vi "UHR-Fleezers Control (host) - Lorentz v2.vi"() -> ()   [LabVIEW 2014] (continued)
        n3462 = call-poly <vilib>:"Mean.vi"("X"=w5310) -> ("mean"=w5257:dbl)  [unwired: 1 out]
        n3463 = call-poly <vilib>:"Mean.vi"("X"=w5266) -> ("mean"=w5250:dbl)  [unwired: 1 out]
        n3464 = call-poly <vilib>:"Mean.vi"("X"=w5268) -> ("mean"=w5255:dbl)  [unwired: 1 out]
        n3465 = call-poly <vilib>:"Mean.vi"("X"=w5267) -> ("mean"=w5253:dbl)  [unwired: 1 out]
        n3466 = Initialize Array(1.0 ("element"), w5238) -> (w5234:dbl[])
        n3467 = Initialize Array(1.0 ("element"), w5219) -> (w5215:dbl[])
        n3468 = Initialize Array(1.0 ("element"), w5260) -> (w5251:dbl[])
        n3469 = Multiply(x=w5234, y=w5235) -> (x*y=w5236:dbl[])
        n3470 = Multiply(x=w5215, y=w5216) -> (x*y=w5217:dbl[])
        n3471 = Multiply(x=w5251, y=w5257) -> (x*y=w5258:dbl[])
        n3472 = Multiply(x=w5251, y=w5253) -> (x*y=w5254:dbl[])
        n3473 = Multiply(x=w5251, y=w5255) -> (x*y=w5256:dbl[])
        n3474 = Multiply(x=w5251, y=w5250) -> (x*y=w5252:dbl[])
        n3475 = Build Array (concatenate)(w5244, w5236) -> (w5246:dbl[])
        n3476 = Build Array (concatenate)(w5225, w5217) -> (w5227:dbl[])
        n3477 = Build Array (concatenate)(w5310, w5258) -> (w5319:dbl[])
        n3478 = Build Array (concatenate)(w5266, w5252) -> (w5314:dbl[])
        n3479 = Build Array (concatenate)(w5268, w5256) -> (w5318:dbl[])
        n3480 = Build Array (concatenate)(w5267, w5254) -> (w5317:dbl[])
        n3481 = Reshape Array(w5246, w5200, w5201) -> (w5242:dbl[][])
        n3482 = Reshape Array(w5227, w5200, w5201) -> (w5223:dbl[][])
        n3483 = Reshape Array(w5319, w5200, w5201) -> (w5297:dbl[][])
        n3484 = Reshape Array(w5314, w5200, w5201) -> (w5280:dbl[][])
        n3485 = Reshape Array(w5318, w5200, w5201) -> (w5272:dbl[][])
        n3486 = Reshape Array(w5317, w5200, w5201) -> (w5287:dbl[][])
        n3487 = Array Subset(array=w5242, index (col)=0 ("index"), length (col)=w5199) -> (w5241:dbl[][])  [unwired: 2 in]
        n3488 = Array Subset(array=w5242, index (col)=w5199) -> (w5239:dbl[][])  [unwired: 3 in]
        n3489 = Array Subset(array=w5223, index (col)=0 ("index"), length (col)=w5199) -> (w5222:dbl[][])  [unwired: 2 in]
        n3490 = Array Subset(array=w5223, index (col)=w5199) -> (w5220:dbl[][])  [unwired: 3 in]
        n3491 = Array Subset(array=w5287, index (col)=0 ("index"), length (col)=w5199) -> (w5292:dbl[][])  [unwired: 2 in]
        n3492 = Array Subset(array=w5287, index (col)=w5199) -> (w5290:dbl[][])  [unwired: 3 in]
        n3493 = Array Subset(array=w5297, index (col)=0 ("index"), length (col)=w5199) -> (w5296:dbl[][])  [unwired: 2 in]
        n3494 = Array Subset(array=w5297, index (col)=w5199) -> (w5294:dbl[][])  [unwired: 3 in]
        n3495 = Array Subset(array=w5272, index (col)=0 ("index"), length (col)=w5199) -> (w5278:dbl[][])  [unwired: 2 in]
        n3496 = Array Subset(array=w5272, index (col)=w5199) -> (w5276:dbl[][])  [unwired: 3 in]
        n3497 = Array Subset(array=w5280, index (col)=0 ("index"), length (col)=w5199) -> (w5285:dbl[][])  [unwired: 2 in]
        n3498 = Array Subset(array=w5280, index (col)=w5199) -> (w5283:dbl[][])  [unwired: 3 in]
        n3499 = for {
          tunnel: w5241 -> [w5328] mode=indexing
          tunnel: [w5327] -> w5240 mode=indexing
          workers-P: _ -> [_]
          n3500 = Reverse 1D Array(array=w5328) -> (reversed array=w5327:dbl[])
        }
        n3501 = for {
          tunnel: w5222 -> [w5326] mode=indexing
          tunnel: [w5325] -> w5221 mode=indexing
          workers-P: _ -> [_]
          n3502 = Reverse 1D Array(array=w5326) -> (reversed array=w5325:dbl[])
        }
        n3503 = for {
          tunnel: w5292 -> [w5334] mode=indexing
          tunnel: [w5333] -> w5291 mode=indexing
          workers-P: _ -> [_]
          n3504 = Reverse 1D Array(array=w5334) -> (reversed array=w5333:dbl[])
        }
        n3505 = for {
          tunnel: w5296 -> [w5336] mode=indexing
          tunnel: [w5335] -> w5295 mode=indexing
          workers-P: _ -> [_]
          n3506 = Reverse 1D Array(array=w5336) -> (reversed array=w5335:dbl[])
        }
        n3507 = for {
          tunnel: w5278 -> [w5330] mode=indexing
          tunnel: [w5329] -> w5277 mode=indexing
          workers-P: _ -> [_]
          n3508 = Reverse 1D Array(array=w5330) -> (reversed array=w5329:dbl[])
        }
        n3509 = for {
          tunnel: w5285 -> [w5332] mode=indexing
          tunnel: [w5331] -> w5284 mode=indexing
          workers-P: _ -> [_]
          n3510 = Reverse 1D Array(array=w5332) -> (reversed array=w5331:dbl[])
        }
        n3511 = Index Array(array=w5297, index (row)=0) -> (element=→"Waveform Graph":dbl[])  [unwired: 1 in]
        n3512 = Add(x=w5240, y=w5239) -> (x+y=w5232:dbl[][])
        n3513 = Add(x=w5221, y=w5220) -> (x+y=w5213:dbl[][])
        n3514 = Add(x=w5291, y=w5290) -> (x+y=w5289:dbl[][])
        n3515 = Add(x=w5295, y=w5294) -> (x+y=w5271:dbl[][])
        n3516 = Add(x=w5277, y=w5276) -> (x+y=w5275:dbl[][])
        n3517 = Add(x=w5284, y=w5283) -> (x+y=w5282:dbl[][])
        n3518 = Divide(x=w5275, y=2) -> (x/y=w5273:dbl[][])
        n3519 = Divide(x=w5289, y=2) -> (x/y=w5179:dbl[][])
        n3520 = To Single Precision Float(number=w5271) -> (single precision float=w5192:sgl[][])
        n3521 = To Single Precision Float(number=w5232) -> (single precision float=w5175:sgl[][])
        n3522 = To Single Precision Float(number=w5213) -> (single precision float=w5168:sgl[][])
        n3523 = Divide(x=w5282, y=2) -> (x/y=w5181:dbl[][])
        n3524 = Transpose 2D Array(2D array=w5273) -> (transposed array=→"Data map":dbl[][])
        n3525 = To Single Precision Float(number=w5179) -> (single precision float=w5185:sgl[][])
        n3526 = To Single Precision Float(number=w5181) -> (single precision float=w5182:sgl[][])
        n3527 = call "IMAQ ArrayToImage"("Image Pixels (Float)"=w5192, "Image"=w5230) -> ("Image Out"=w5194:T2)  [unwired: 8 in, 1 out]
        n3528 = call "IMAQ ArrayToImage"("Image Pixels (Float)"=w5175, "Image"=w5229) -> ("Image Out"=w5177:T2)  [unwired: 8 in, 1 out]
        n3529 = call "IMAQ ArrayToImage"("Image Pixels (Float)"=w5168, "Image"=w5210) -> ("Image Out"=w5170:T2)  [unwired: 8 in, 1 out]
        n3530 = call "IMAQ ArrayToImage"("Image Pixels (Float)"=w5185, "Image"=w5211) -> ("Image Out"=w5187:T2)  [unwired: 8 in, 1 out]
        n3531 = call "IMAQ Symmetry"("Type of Symmetry"=w5193, "Image Src"=w5194) -> ("Image Dst Out"=w5190:T2)  [unwired: 3 in, 1 out]
        n3532 = call "IMAQ ArrayToImage"("Image Pixels (Float)"=w5182, "Image"=w5212) -> ("Image Out"=w5184:T2)  [unwired: 8 in, 1 out]
        n3533 = call "IMAQ Symmetry"("Type of Symmetry"=w5176, "Image Src"=w5177) -> ("Image Dst Out"=w5173:T2)  [unwired: 3 in, 1 out]
        n3534 = call "IMAQ Symmetry"("Type of Symmetry"=w5169, "Image Src"=w5170) -> ("Image Dst Out"=w5166:T2)  [unwired: 3 in, 1 out]
        n3535 = call "IMAQ Symmetry"("Type of Symmetry"=w5186, "Image Src"=w5187) -> ("Image Dst Out"=→"Detection Laser X":T2)  [unwired: 3 in, 1 out]
        n3536 = call "IMAQ Symmetry"("Type of Symmetry"=w5183, "Image Src"=w5184) -> ("Image Dst Out"=→"Detection Laser Y":T2)  [unwired: 3 in, 1 out]
        n3537 = call "IMAQ Set Simple Calibration"("Calibration Axis Info"=T52 {"Origin Pixel"={"X"=0.0, "Y"=0.0}, "Angle Relative to Horizontal (deg)"=0.0, "Axis Reference"=0}, "Grid Descriptor"=T53 {"X Step"=0.3, "Y Step"=0.3, "Unit"=enum."Undefined"}, "Image"=w5190) -> ("Calibrated Image"=→"APD 1":T2)  [unwired: 7 in, 1 out]
        n3538 = call "IMAQ Set Simple Calibration"("Calibration Axis Info"=T52 {"Origin Pixel"={"X"=0.0, "Y"=0.0}, "Angle Relative to Horizontal (deg)"=0.0, "Axis Reference"=0}, "Grid Descriptor"=T53 {"X Step"=0.3, "Y Step"=0.3, "Unit"=enum."Undefined"}, "Image"=w5173) -> ("Calibrated Image"=→"APD 2":T2)  [unwired: 7 in, 1 out]
        n3539 = call "IMAQ Set Simple Calibration"("Calibration Axis Info"=T52 {"Origin Pixel"={"X"=0.0, "Y"=0.0}, "Angle Relative to Horizontal (deg)"=0.0, "Axis Reference"=0}, "Grid Descriptor"=T53 {"X Step"=0.3, "Y Step"=0.3, "Unit"=enum."Undefined"}, "Image"=w5166) -> ("Calibrated Image"=→"APD 3":T2)  [unwired: 7 in, 1 out]
      }
    }
    n3540 = case "For computing FFTs for display" shown="True" "Compute FFT" {
      tunnel: w4647 -> [_ w5808]
      frame False {
      }
      frame True {
        n3541 = Build Array("FFT 1 Choice 1", "FFT 1 Choice 2", "FFT 2 Choice 1", "FFT 2 Choice 2") -> (w5801:u16[])
        n3542 = Array Size(array=w5808) -> (size(s)=w5807:i32)
        n3543 = feedback-in #20(w5801) -> ()
        n3544 = feedback #20(u16[] [100, 100, 100, 100]) -> (w5802:u16[])
        n3545 = feedback-in #21("# Spectra to Ave.") -> ()
        n3546 = feedback #21("# Spectra to Ave.") -> (w5799:dbl)
        n3547 = Not Equal?(x="# Spectra to Ave.", y=w5799) -> (x != y?=w5798:bool)
        n3548 = Not Equal?(x=w5801, y=w5802) -> (x != y?=w5800:bool)
        n3549 = feedback #22(1.0) -> (w5785:dbl)
        n3550 = Compound Arithmetic op=OR("Reset FFT", w5800, w5798) -> (w5783:bool)
        n3551 = Select(t=1.0, s=w5783, f=w5785) -> (s? t:f=w5787:dbl)
        n3552 = Greater?(x=w5787, y="# Spectra to Ave.") -> (0:w5806:bool)
        n3553 = Increment(x=w5787) -> (x+1=w5786:dbl)
        n3554 = feedback-in #22(w5786) -> ()
        n3555 = local read "DMA Update Period (s)"() -> (w5781:dbl)
        n3556 = Multiply(x="# Spectra to Ave.", y=w5781) -> (x*y=→"Ave. Time (s)":dbl)
        n3557 = Build Array(cluster{"f0":dbl, "df":dbl, "magnitude":dbl[]} {"f0"=0.0, "df"=0.0, "magnitude"=[]} ("PSD")) -> (w5790:cluster{"f0":dbl, "df":dbl, "magnitude":dbl[]}[])
        n3558 = Build Array(w5790, w5790, w5790, w5790) -> (w5792:T62)
        n3559 = feedback #23(w5792) -> (w5797:T62)
        n3560 = for {
          N: 4 -> [_]
          tunnel: w5801 -> [w5830] mode=indexing
          tunnel: w5808 -> [w5831]
          tunnel: w5807 -> [w5833]
          tunnel: w5783 -> [w5826]
          tunnel: w5806 -> [w5825]
          tunnel: "# Spectra to Ave." -> [w5824]
          tunnel: [w5823] -> w5796 mode=indexing
          tunnel: w5797 -> [w5828] mode=indexing
          tunnel: [w5827] -> w5784 mode=indexing
          tunnel: w5787 -> [w5822]
          n3561 = Less?(x=w5830, y=w5833) -> (x < y?=w5832:bool)
          n3562 = Index Array(array=w5831, index=w5830) -> (element=w5829:waveform(dbl))
          n3563 = case shown="True" w5832 {
            tunnel: w5829 -> [_ w5850]
            tunnel: w5828 -> [w5835 w5848]
            tunnel: [w5835 w5836] -> w5827
            tunnel: w5826 -> [_ w5847]
            tunnel: w5825 -> [_ w5840]
            tunnel: w5824 -> [_ w5839]
            tunnel: [cluster{"f0":dbl, "df":dbl, "magnitude":dbl[]} {"f0"=0.0, "df"=0.0, "magnitude"=[]} ("PSD") w5841] -> w5823
            tunnel: w5822 -> [_ w5838]
            frame False {
            }
            frame True {
              n3564 = call <vilib>:"Std Deviation and Variance.vi"("X"=w5850) -> ("mean"=w5851:dbl)  [unwired: 1 in, 2 out]
              n3565 = Subtract(x=w5850, y=w5851) -> (x-y=w5849:waveform(dbl))
              n3566 = xnode "Spectral Measurements"("Signals"=w5849) -> ("PSD"=w5843:cluster{"f0":dbl, "df":dbl, "magnitude":dbl[]})  [unwired: 1 in, 1 out]
              n3567 = case shown="False" w5847 {
                tunnel: w5848 -> [w5860 _]
                tunnel: [w5856 w5865] -> w5836
                tunnel: w5843 -> [w5859 w5866]
                tunnel: w5840 -> [w5858 _]
                frame False {
                  n3568 = Build Array (concatenate)(w5860, w5859) -> (w5857:cluster{"f0":dbl, "df":dbl, "magnitude":dbl[]}[])
                  n3569 = case shown="True" w5858 {
                    tunnel: w5857 -> [w5861 w5864]
                    tunnel: [w5861 w5862] -> w5856
                    frame False {
                    }
                    frame True {
                      n3570 = Delete From Array(array=w5864, index=0) -> (array with subset deleted=w5862:cluster{"f0":dbl, "df":dbl, "magnitude":dbl[]}[])  [unwired: 1 in, 1 out]
                    }
                  }
                }
                frame True {
                  n3571 = Build Array(w5866) -> (w5865:cluster{"f0":dbl, "df":dbl, "magnitude":dbl[]}[])
                }
              }
              n3572 = for {
                tunnel: w5836 -> [w5855] mode=indexing
                tunnel: [w5854] -> w5846 mode=indexing
                workers-P: _ -> [_]
                n3573 = Unbundle By Name(w5855) -> ("magnitude"=w5854:dbl[])
              }
              n3574 = Transpose 2D Array(2D array=w5846) -> (transposed array=w5845:dbl[][])
              n3575 = for {
                tunnel: w5845 -> [w5853] mode=indexing
                tunnel: [w5852] -> w5844 mode=indexing
                workers-P: _ -> [_]
                n3576 = Add Array Elements(numeric array=w5853) -> (sum=w5852:dbl)
              }
              n3577 = Select(t=w5839, s=w5840, f=w5838) -> (s? t:f=w5837:dbl)
              n3578 = Divide(x=w5844, y=w5837) -> (x/y=w5842:dbl[])
              n3579 = Bundle By Name(cluster=w5843, "magnitude"=w5842) -> (w5841:cluster{"f0":dbl, "df":dbl, "magnitude":dbl[]})
            }
          }
        }
        n3580 = case shown="True" w5783 {
          tunnel: w5784 -> [w5815 w5821]
          tunnel: [w5815 w5816] -> w5782
          frame False {
          }
          frame True {
            n3581 = Array Subset(array=w5821, index (row)=0 ("index"), length (row)=4 ("length"), index (col)=0 ("index"), length (col)=1 ("length")) -> (w5816:T62)
          }
        }
        n3582 = feedback-in #23(w5782) -> ()
        n3583 = Split 1D Array(array=w5796, index=2) -> (first subarray=→"FFT 1":cluster{"f0":dbl, "df":dbl, "magnitude":dbl[]}[], second subarray=→"FFT 2":cluster{"f0":dbl, "df":dbl, "magnitude":dbl[]}[])
      }
    }
    n3584 = local read "Offset Values"() -> (w4394:T17)
    n3585 = local read "T1 calibration"() -> (w4452:T6)
    n3586 = local read "T2 calibration"() -> (w4451:T5)
    n3587 = call-poly <vilib>:"Index Waveform Array.vi"("index"=16, "waveform array"=w4426) -> ("waveform"=w4425:waveform(dbl))  [unwired: 8 in, 1 out]
    n3588 = Unbundle By Name(w4441) -> ("Y"=w4450:dbl[])
    n3589 = Unbundle By Name(w4438) -> ("Y"=w4449:dbl[])
    n3590 = local read "Offset file step size"() -> (w4391:dbl)
    n3591 = Unbundle By Name(w4425) -> ("Y"=→"PSD Y Sum":dbl[])
    n3592 = call "calibrate trap data V2.vi"("Offset File step size"=w4391, "delta frequency"=w4393, "Dynamic offset update"="Dynamic offset\nupdate", "Offsets"=w4394, "T2 cal"=w4451, "T2"=w4449, "T1 cal"=w4452, "T1"=w4450) -> ("T2 force (pN)"=w4442:dbl[], "T2 position (nm)"=w4443:dbl[], "T1 force (pN)"=w4444:dbl[], "T1 position (nm)"=w4445:dbl[])
    n3593 = Bundle By Name(cluster=w4441, "Y"=w4445) -> (w4440:waveform(dbl))
    n3594 = Bundle By Name(cluster=w4441, "Y"=w4444) -> (w4439:waveform(dbl))
    n3595 = Bundle By Name(cluster=w4438, "Y"=w4443) -> (w4437:waveform(dbl))
    n3596 = Bundle By Name(cluster=w4438, "Y"=w4442) -> (w4436:waveform(dbl))
    n3597 = Subtract(x=w4445, y=w4443) -> (x-y=w4690:dbl[])
    n3598 = case shown="True" "Read Lateness and Rel Phase" {
      tunnel: w4400 -> [w5112 w5145]
      tunnel: w4522 -> [w5113 w5144]
      tunnel: [w5112 w5117] -> w4688
      tunnel: [w5113 w5116] -> w4687
      frame False {
      }
      frame True {
        n3599 = xnode "Read/Write Control"("FPGA VI Reference In"=w5145, "error in"=w5144) -> ("FPGA VI Reference Out"=w5119:T31, "error out"=w5118:errorcluster, "GI Relative phase"=→"GI relative phase":i16, "Relative phase"=→"Relative phase (AI1)":i16, "AI Late Counter"=→"Late Counter (AI1)":u8, "GI Late Counter"=→"GI Late Counter":u8, "MCL Late Counter"=→"MCL Late Counter":u8, "MCL Relative Phase"=→"Relative Phase (MCL)":i16, "APD Acq Relative Phase"=→"APD Acq Relative Phase":i16, "APD 1 Gate Relative Phase"=→"APD 1 Gate Relative Phase":i16, "APD 2 Gate Relative Phase"=→"APD 2 Gate Relative Phase":i16, "APD Acq Late Counter"=→"APD Acq Late Counter":u8, "APD 1 Gate Late Counter"=→"APD 1 Gate Late Counter":u8, "APD 2 Gate Late Counter"=→"APD 2 Gate Late Counter":u8, "Green FB Relative Phase"=→"Relative phase (Green FB)":i16, "GI Relative phase 2"=→"GI relative phase 2":i16, "GI Late Counter 2"=→"GI Late Counter 2":u8, "Trap Pos FIFO Timeout"=→"Trap Pos FIFO Timeout":u16, "Trap AI FIFO Timeout"=→"Trap AI FIFO Timeout":u16, "RI Late Counter"=→"RI Late Counter":u8, "RI Relative phase"=→"RI relative phase":i16, "Green Late Counter"=→"Green AI Late Counter":u8, "BI Late Counter (AO)"=→"Late Counter (BI AO)":u8, "Blue Late Counter (D)"=→"Late Counter (BI DO)":u8, "BI Relative phase (AO)"=→"Relative phase (BI AO)":i16, "BI Relative phase (D)"=→"Relative phase (BI DO)":i16)
        n3600 = xnode "Read/Write Control"("FPGA VI Reference In"=w5119, "error in"=w5118) -> ("FPGA VI Reference Out"=w5117:T31, "error out"=w5116:errorcluster, "APD 3 Gate Late Counter"=→"APD 3 Gate Late Counter":u8, "APD 3 Gate Relative Phase"=→"APD 3 Gate Relative Phase":i16)
      }
    }
    n3601 = Negate(x=w4690) -> (-x=w4506:dbl[])
    n3602 = Subtract(x=w4506, y="Offset (nm)") -> (x-y=w4665:dbl[])
    n3603 = case "Choose calibrated display" shown="2" "Calibration" {
      tunnel: w4441 -> [w5147 _ _]
      tunnel: w4438 -> [w5146 _ _]
      tunnel: [w5147 w5149 w5151] -> w4417
      tunnel: [w5146 w5148 w5150] -> w4701
      tunnel: w4440 -> [_ w5149 _]
      tunnel: w4439 -> [_ _ w5151]
      tunnel: w4437 -> [_ w5148 _]
      tunnel: w4436 -> [_ _ w5150]
      frame 0, Default {
      }
      frame 1 {
      }
      frame 2 {
      }
    }
    n3604 = Bundle By Name(cluster=w4441, "Y"=w4665) -> (w4435:waveform(dbl))
    "Bead Separation" <- w4435
    n3605 = feedback #24(w4665) -> (w4664:dbl[])
    n3606 = Build Array (concatenate)(w4665, w4664) -> (w4447:dbl[])
    n3607 = Split 1D Array(array=w4447, index=w4564) -> (first subarray=w4448:dbl[])  [unwired: 1 out]
    n3608 = feedback-in #24(w4448) -> ()
    n3609 = Build Array(w4441, w4440, w4439, w4438, w4437, w4436, w4435) -> (w4434:waveform(dbl)[])
    n3610 = Not(x="Trap Trig. Fl.") -> (.not. x?=w4540:bool)
    n3611 = Unbundle By Name(w4417) -> ("Y"=w4507:dbl[])
    n3612 = Unbundle By Name(w4701) -> ("Y"=w4666:dbl[])
    n3613 = call-poly <vilib>:"Mean.vi"("X"=w4448) -> ("mean"=w4661:dbl)  [unwired: 1 out]
    "Bead Mean (nm)" <- w4661
    n3614 = Multiply(x=w4701, y=-1.0) -> (x*y=w4413:waveform(dbl))
    n3615 = call-poly <vilib>:"Mean.vi"("X"=w4507) -> ("mean"=w4510:dbl)  [unwired: 1 out]
    "T1 X" <- w4510
    n3616 = call-poly <vilib>:"Mean.vi"("X"=w4666) -> ("mean"=w4509:dbl)  [unwired: 1 out]
    "T2 X" <- w4509
    n3617 = Subtract(x=w4448, y=w4661) -> (x-y=w4660:dbl[])
    n3618 = Add(1:w4413, 2:w4417) -> (0:w4416:waveform(dbl))  [unwired: 1 in, 1 out]
    n3619 = Square(x=w4660) -> (x^2=w4659:dbl[])
    n3620 = Divide(x=w4416, y=2.0) -> (x/y=w4414:waveform(dbl))
    n3621 = Negate(x=w4666) -> (-x=w4460:dbl[])
    n3622 = call-poly <vilib>:"Mean.vi"("X"=w4659) -> ("mean"=w4658:dbl)  [unwired: 1 out]
    n3623 = Negate(x=w4509) -> (-x=w4508:dbl)
    n3624 = Square Root(x=w4658) -> (sqrt(x)=w4657:dbl)
    n3625 = Add(x=w4507, y=w4460) -> (x+y=w4667:dbl[])
    n3626 = Add(x=w4510, y=w4508) -> (x+y=w4696:dbl)
    n3627 = Multiply(x=10.0, y=w4657) -> (x*y=→"RMS (Ang)":dbl)
    n3628 = Divide(x=w4667, y=2.0) -> (x/y=w4463:dbl[])
    n3629 = Subtract(x=w4510, y=w4508) -> (x-y=→"Difference":dbl)
    n3630 = Build Array(w4417, w4413, w4414) -> (→"Force":waveform(dbl)[])
    n3631 = Select(t=w4460, s="Only check fixed trap T2", f=w4463) -> (s? t:f=→"Vec Mean of T1 T2":dbl[])
    n3632 = Divide(x=w4696, y=2.0) -> (x/y=w4388:dbl)
    "Mean" <- w4388
    n3633 = feedback-in #25("Trap Trig. Fl.") -> ()
    n3634 = feedback #25("Trap Trig. Fl.") -> (w4538:bool)
    n3635 = And(x=w4540, y=w4538) -> (x .and. y?=w4539:bool)
    n3636 = case "If have just turned off triggering" shown="True" w4539 {
      tunnel: w4401 -> [_ w4947]
      tunnel: w4522 -> [_ w4946]
      frame False {
      }
      frame True {
        w4945 = FALSE ("FPGA Trap Trig")
        n3637 = xnode "Read/Write Control"("FPGA VI Reference In"=w4947, "error in"=w4946, "FPGA Trap Trig"=w4945) -> ("FPGA VI Reference Out"=w4944:T31, "error out"=w4943:errorcluster)
        n3638 = xnode "Read/Write Control"("FPGA VI Reference In"=w4944, "error in"=w4943, "TTrig?"=w4945) -> ()  [unwired: 2 out]
        n3639 = local write "Initializing"(FALSE ("Initializing")) -> ()
        n3640 = local write "Triggered"(FALSE ("Triggered")) -> ()
        n3641 = local write "Waiting"(FALSE ("Waiting")) -> ()
      }
    }
    n3642 = Not(x=w4538) -> (.not. x?=w4551:bool)
    n3643 = And(x="Trap Trig. Fl.", y=w4551) -> (x .and. y?=w4548:bool)
    n3644 = Or(x=w4548, y="Reinitialize") -> (x .or. y?=w4534:bool)
    n3645 = feedback #26(w4544) -> (w4549:string)
    n3646 = Select(t=w4544, s=w4548, f=w4549) -> (s? t:f=w4543:string)
    n3647 = Select(t=w4544, s="Reinitialize", f=w4543) -> (s? t:f=w4542:string)
    n3648 = local read "Tether"() -> (w4669:bool)
    n3649 = feedback #27(0) -> (w4546:i32)
    n3650 = case "For determining if there is a tether still" shown="True" w4669 {
      tunnel: w4388 -> [_ w5071]
      frame False {
      }
      frame True {
        n3651 = Greater?(x="Lost Tether Alarm Threshold (pN)", y=w5071) -> (0:w5069:bool)
        n3652 = case shown="True" w5069 {
          frame False {
          }
          frame True {
            w5072 = FALSE ("Value (Signaling)")
            n3653 = flat-sequence {
              frame #0 {
                # "stop only if saving"
                n3654 = local read "Saving..."() -> (w5084:bool)
                n3655 = And(x=w5084, y="TA Cancel Save?") -> (x .and. y?=w5083:bool)
                n3656 = local write "Stop Saving"(w5083) -> ()
              }
              frame #1 {
                n3657 = case shown="True" "TA Green Off?" {
                  frame False {
                  }
                  frame True {
                    w5087 = FALSE ("Fl. Triggered...")
                    n3658 = local write "Fl. Triggered..."(w5087) -> ()
                    n3659 = property on="Green Laser ON" class="Bool (strict)"("Val(Sgnl)"=w5087) -> ()  [unwired: 2 in, 2 out]
                  }
                }
              }
            }
            n3660 = local read "Time tether formed"() -> (w5078:timestamp)
            n3661 = Get Date/Time In Seconds() -> (seconds since 1Jan1904=w5079:timestamp)
            n3662 = Subtract(x=w5079, y=w5078) -> (x-y=w5077:dbl)
            n3663 = Number To Decimal String(number=w5077) -> (decimal integer string=w5074:string)  [unwired: 1 out]
            n3664 = local read "Messages"() -> (w5081:string)
            n3665 = call <vilib>:"Beep.vi"() -> ()  [unwired: 3 in, 9 out]
            n3666 = Concatenate Strings("Lost tether (" ("Message to add"), w5074, " s)." ("string")) -> (w5076:string)
            n3667 = local write "Tether"(FALSE ("Tether")) -> ()
            n3668 = call "Update messages.vi"("Message to add"=w5076, "Old message string"=w5081) -> ("New message string"=w5080:string)
            n3669 = local write "Messages"(w5080) -> ()
            n3670 = property on="Fl. Triggered..." class="Bool (strict)"("Val(Sgnl)"=w5072) -> ()  [unwired: 2 in, 2 out]
            n3671 = local write "Dip for Protein"(w5072) -> ()
            n3672 = property on="Trap Pos. FB ON" class="Bool (strict)"("Val(Sgnl)"=w5072) -> ()  [unwired: 2 in, 2 out]
            n3673 = property on="Trap Trig. Fl." class="Bool (strict)"("Val(Sgnl)"=w5072) -> ()  [unwired: 2 in, 2 out]
          }
        }
      }
    }
    n3674 = case "For triggering actions based on the trap position (e.g., turning the excitation laser on if trap under feedback moves so far)" shown="True" "Trap Trig. Fl." {
      tunnel: w4530 -> [_ w4960]
      tunnel: w4542 -> [_ w4959]
      tunnel: ["" ("t") w4958] -> w4550
      tunnel: w4534 -> [_ w4957]
      tunnel: [0 ("t") w4956] -> w4547
      tunnel: w4546 -> [_ w4955]
      tunnel: w4401 -> [_ w4954]
      tunnel: w4522 -> [_ w4953]
      frame False {
      }
      frame True {
        n3675 = case shown="\"Wait for trigger\"" w4959 {
          tunnel: w4960 -> [w4977 _ _ w5025]
          tunnel: [w4974 w5006 "" ("t") w5028] -> w4958
          tunnel: w4957 -> [_ _ _ w5016]
          tunnel: [w4973 w5003 0 ("t") w5017] -> w4956
          tunnel: w4955 -> [_ w5005 _ w5023]
          tunnel: w4954 -> [w4962 w5000 _ w5019]
          tunnel: w4953 -> [w4961 w4999 _ w5018]
          frame "Wait for trigger" {
            n3676 = local read "Trap Trig. (FPGA)"() -> (w4965:bool)
            n3677 = Subtract(x=w4977, y="Mean T1 Position\nto compare (nm)") -> (x-y=w4970:dbl[])
            n3678 = call <vilib>:"Std Deviation and Variance.vi"("X"=w4970) -> ("mean"=→"mean":dbl, "standard deviation"=→"standard\ndeviation":dbl)  [unwired: 1 in, 1 out]
            n3679 = Array Max & Min(array=w4970) -> (max value=→"max value":dbl, min value=→"min value":dbl)  [unwired: 2 out]
            n3680 = Greater?(x=w4970, y="Threshold (nm)") -> (0:w4980:bool[])
            n3681 = case shown="True" w4965 {
              tunnel: w4962 -> [_ w4986]
              tunnel: w4961 -> [_ w4985]
              tunnel: [FALSE ("TTrig?") w4984] -> w4968
              frame False {
              }
              frame True {
                n3682 = xnode "Read/Write Control"("FPGA VI Reference In"=w4986, "error in"=w4985) -> ("TTrig?"=w4984:bool)  [unwired: 2 out]
              }
            }
            n3683 = Or Array Elements(Boolean array=w4980) -> (logical OR=w4967:bool)
            n3684 = Select(t=w4968, s=w4965, f=w4967) -> (s? t:f=w4966:bool)
            n3685 = Not(x=w4965) -> (.not. x?=w4964:bool)
            n3686 = And(x=w4966, y=w4964) -> (x .and. y?=w4963:bool)
            n3687 = Select(t="Triggered", s=w4966, f="Wait for trigger") -> (s? t:f=w4974:string)
            n3688 = case shown="True" w4966 {
              tunnel: [0 0] -> w4973
              tunnel: w4962 -> [_ w4991]
              tunnel: w4961 -> [_ w4990]
              frame False {
                "Waiting" <- TRUE ("Waiting")
              }
              frame True {
                n3689 = xnode "Read/Write Control"("FPGA VI Reference In"=w4991, "error in"=w4990, "TTrig?"=FALSE) -> ()  [unwired: 2 out]
                n3690 = local read "Messages"() -> (w4994:string)
                n3691 = call <vilib>:"Beep.vi"() -> ()  [unwired: 12 in]
                n3692 = call "Update messages.vi"("Message to add"="Unwinding trigger.", "Old message string"=w4994) -> ("New message string"=w4995:string)
                n3693 = local write "Messages"(w4995) -> ()
                n3694 = local write "Waiting"(FALSE ("Waiting")) -> ()
                "Triggered" <- TRUE ("Triggered")
              }
            }
            n3695 = case "Only need to turn on laser if host triggered" shown="True" w4963 {
              frame False {
              }
              frame True {
                n3696 = property on="Green Laser ON" class="Bool (strict)"("Val(Sgnl)"=TRUE ("Value (Signaling)")) -> ()  [unwired: 2 in, 2 out]
              }
            }
          }
          frame "Triggered" {
            n3697 = local read "Trap Trig. (FPGA)"() -> (w5002:bool)
            n3698 = Increment(x=w5005) -> (x+1=w5003:i32)
            n3699 = Greater Or Equal?(x=w5003, y="Fl. ON time (n)") -> (x >= y?=w5001:bool)
            n3700 = Select(t="Wait for trigger", s=w5001, f="Triggered" ("t")) -> (s? t:f=w5006:string)
            n3701 = And(x=w5001, y=w5002) -> (x .and. y?=w4998:bool)
            n3702 = case shown="True" w4998 {
              tunnel: w5000 -> [_ w5010]
              tunnel: w4999 -> [_ w5009]
              frame False {
              }
              frame True {
                n3703 = xnode "Read/Write Control"("FPGA VI Reference In"=w5010, "error in"=w5009, "FPGA Trap Trig"=TRUE) -> ()  [unwired: 2 out]
              }
            }
            n3704 = case shown="True" w5001 {
              frame False {
              }
              frame True {
                w5012 = FALSE ("Value (Signaling)")
                n3705 = local write "Triggered"(w5012) -> ()
                n3706 = local write "Waiting"(TRUE ("Waiting")) -> ()
                n3707 = property on="Green Laser ON" class="Bool (strict)"("Val(Sgnl)"=w5012) -> ()  [unwired: 2 in, 2 out]
              }
            }
          }
          frame "Do nothing" {
          }
          frame "Initialize", Default {
            n3708 = Increment(x=w5023) -> (x+1=w5027:i32)
            n3709 = Select(t=1, s=w5016, f=w5027) -> (s? t:f=w5017:i32)
            n3710 = feedback #28(w5025) -> (w5031:dbl[])
            n3711 = Build Array (concatenate)(w5025, w5031) -> (w5024:dbl[])
            n3712 = Greater Or Equal?(x=w5017, y="Wait to get offset (n)") -> (x >= y?=w5020:bool)
            n3713 = Select(t=w5025, s=w5016, f=w5024) -> (s? t:f=w5026:dbl[])
            n3714 = feedback-in #28(w5026) -> ()
            n3715 = call-poly <vilib>:"Mean.vi"("X"=w5026) -> ("mean"=w5021:dbl)  [unwired: 1 out]
            n3716 = local write "Mean T1 Position\nto compare (nm)"(w5021) -> ()
            n3717 = case shown="True" w5016 {
              tunnel: w5019 -> [_ w5037]
              tunnel: w5018 -> [_ w5036]
              frame False {
              }
              frame True {
                w5033 = FALSE ("FPGA Trap Trig")
                n3718 = xnode "Read/Write Control"("FPGA VI Reference In"=w5037, "error in"=w5036, "FPGA Trap Trig"=w5033) -> ("FPGA VI Reference Out"=w5035:T31, "error out"=w5034:errorcluster)
                n3719 = xnode "Read/Write Control"("FPGA VI Reference In"=w5035, "error in"=w5034, "TTrig?"=w5033) -> ()  [unwired: 2 out]
              }
            }
            n3720 = Select(t="Wait for trigger", s=w5020, f="Initialize") -> (s? t:f=w5028:string)
            n3721 = case shown="True" w5020 {
              tunnel: w5021 -> [_ w5040]
              tunnel: w5019 -> [_ w5049]
              tunnel: w5018 -> [_ w5048]
              frame False {
                n3722 = local write "Waiting"(FALSE ("Waiting")) -> ()
                "Initializing" <- TRUE ("Initializing")
              }
              frame True {
                n3723 = local read "Threshold (nm)"() -> (w5052:dbl)
                n3724 = local read "AOM X Cal (nm/MHz)"() -> (w5051:dbl)
                n3725 = Add(x=w5040, y=w5052) -> (x+y=w5053:dbl)
                n3726 = Divide(x=w5053, y=w5051) -> (x/y=w5050:dbl)
                n3727 = call "IR AOM freq to word.vi"("Frequency In (MHz)"=w5050) -> ("Frequency Word Out (double)"=w5047:dbl)
                n3728 = local write "Initializing"(FALSE ("Initializing")) -> ()
                n3729 = local write "Waiting"(TRUE ("Waiting")) -> ()
                n3730 = To Quad Integer(1:w5047) -> (0:w5046:i64)
                n3731 = xnode "Read/Write Control"("FPGA VI Reference In"=w5049, "error in"=w5048, "FPGA TTrig Thresh"=w5046) -> ("FPGA VI Reference Out"=w5043:T31, "error out"=w5042:errorcluster)
                n3732 = xnode "Read/Write Control"("FPGA VI Reference In"=w5043, "error in"=w5042, "FPGA Trap Trig"=TRUE) -> ()  [unwired: 2 out]
              }
            }
          }
        }
      }
    }
    n3733 = feedback-in #26(w4550) -> ()
    n3734 = feedback-in #27(w4547) -> ()
    n3735 = xnode ("Read/Write Control")("FPGA VI Reference In"=w4688, "error in"=w4687) -> ("FPGA VI Reference Out"=w4390:T31, "error out"=w4532:errorcluster, "AI2 Y Sum Set 1"=w4757:i16, "AI2 Y Sum Set 2"=w4756:i16, "AI1 X Set 1"=w4596:fxp<+/-,16,1>, "AI1 X Set 2"=w4595:fxp<+/-,16,1>, "Trap Pos FB Int Signal"=→"Trap Pos FB Int Signal":fxp<+/-,24,9>, "Trap Pos FB Int-Norm Signal"=→"Trap Pos FB Int-Norm Signal":fxp<+/-,16,1>, "Trap Pos FB Action"=w4589:i64, "Scanning"=→"AOD Scanning":bool, "Scan I"=→"AOD Scan I":u64, "Scanning MCL"=w4759:bool, "Scan I (MCL)"=→"MCL Scan I":u64, "Green FB Sum"=w4702:i16, "Trap Pos FB Action"=w4521:i64, "TTrig Fin Thresh"=w4517:i64, "Red FB Intensity"=w4501:i16, "Blue Intensity"=w4496:i16, "BD1 Frequency Out 1"=w4418:u64)
    "MCL Scanning" <- w4759
    "Trap Pos FB Action" <- w4589
    n3736 = Divide(x=w4501, y=3276.7) -> (x/y=w4500:dbl)
    "Red laser intensity (V)" <- w4500
    n3737 = Divide(x=w4496, y=3276.7) -> (x/y=w4495:dbl)
    "Blue laser intensity (V)" <- w4495
    n3738 = Divide(x=w4702, y=3276.7) -> (x/y=w4499:dbl)
    "Green laser intensity (V)" <- w4499
    n3739 = local read "FB Trig Integrate"() -> (w4515:u32)
    n3740 = Divide(x=w4521, y=w4515) -> (x/y=w4514:dbl)
    "TTrig Sig (Int)" <- w4514
    n3741 = Bundle(w4499, w4500, w4495) -> (→"Fluorescence laser intensities plot":cluster{dbl, dbl, dbl})  [unwired: 1 in]
    n3742 = Divide(x=w4517, y=w4515) -> (x/y=w4512:dbl)
    "TTrig Fin Thresh (Int)" <- w4512
    n3743 = local read "AOM X Cal (nm/MHz)"() -> (w4520:dbl)
    n3744 = local read "AI2 (V)"() -> (w4758:cluster{"Set 1":dbl, "Set 2":dbl})
    n3745 = Bundle By Name(cluster=w4758, "Set 1"=w4757, "Set 2"=w4756) -> (w4420:cluster{"Set 1":dbl, "Set 2":dbl})
    n3746 = Divide(x=w4589, y=327.67) -> (x/y=→"Action (%)":dbl)
    n3747 = case shown="True" "Semi Passive Mode" {
      tunnel: w4388 -> [_ w4783]
      frame False {
      }
      frame True {
        n3748 = local read "Target Force (pN)"() -> (w4781:dbl)
        n3749 = Less?(x="Jump Force (pN)", y=w4781) -> (x < y?=w4779:bool)
        n3750 = case shown="False" w4779 {
          tunnel: "Jump Force (pN)" -> [w4789 w4792]
          tunnel: w4783 -> [w4788 w4791]
          tunnel: [w4787 w4790] -> w4782
          frame False {
            n3751 = Less?(x=w4789, y=w4788) -> (x < y?=w4787:bool)
          }
          frame True {
            n3752 = Greater?(x=w4792, y=w4791) -> (0:w4790:bool)
          }
        }
        n3753 = case shown="False" w4782 {
          frame False {
            n3754 = local read "Trap Pos. FB ON"() -> (w4784:bool)
            n3755 = case shown="False" w4784 {
              frame False {
              }
              frame True {
                n3756 = property on="Trap Pos. FB ON" class="Bool (strict)"("Val(Sgnl)"=FALSE) -> ()  [unwired: 2 in, 2 out]
              }
            }
          }
          frame True {
            n3757 = property on="Trap Pos. FB ON" class="Bool (strict)"("Val(Sgnl)"=TRUE) -> ()  [unwired: 2 in, 2 out]
          }
        }
      }
    }
    n3758 = local read "Trap X (AI1)"() -> (w4609:T12)
    n3759 = call "IR AOM word double to freq.vi"("Frequency Word In (double)"=w4512) -> ("Frequency Out (MHz)"=w4511:dbl)
    n3760 = call "IR AOM word double to freq.vi"("Frequency Word In (double)"=w4514) -> ("Frequency Out (MHz)"=w4513:dbl)
    n3761 = Divide(x=w4420, y=3276.7) -> (x/y=w4754:cluster{"Set 1":dbl, "Set 2":dbl})
    n3762 = Multiply(x=w4513, y=w4520) -> (x*y=w4519:dbl)
    "TTrig Sig (nm)" <- w4519
    n3763 = Multiply(x=w4511, y=w4520) -> (x*y=w4518:dbl)
    "TTrig Fin Thresh (nm)" <- w4518
    n3764 = local write "AI2 (V)"(w4754) -> ()
    n3765 = Bundle(cluster=w4609, "Trap 1"=w4596, "Trap 2"=w4595) -> (→"Trap X (AI1)":T12)
    n3766 = local read "Trap Pos. FB ON"() -> (w4395:bool)
    n3767 = local read "Dynamic Force FB (ronen)"() -> (w4396:bool)
    n3768 = Bundle(w4519, w4518) -> (→"TTrig":cluster{dbl, dbl})  [unwired: 1 in]
    n3769 = Compound Arithmetic op=AND(w4396, "Real time Offset file correction for setpoint", w4395) -> (w4397:bool)
    n3770 = case shown="True" w4397 {
      tunnel: w4418 -> [_ _]
      tunnel: w4393 -> [_ w4811]
      tunnel: w4390 -> [_ w4794]
      frame False {
      }
      frame True {
        # "Changed by Ronen - real time update of set point\naccording to offset file"
        n3771 = local read "T1 calibration"() -> (w4806:T6)
        n3772 = local read "Offset file step size"() -> (w4813:dbl)
        n3773 = local read "Setpoint offset\ncorrection values"() -> (w4810:dbl[])
        n3774 = Multiply(x="Target Force (pN)", y=2.0) -> (x*y=w4807:dbl)
        n3775 = local read "Negate Diff?"() -> (w4795:bool)
        n3776 = Unbundle By Name(w4806) -> ("T1 alpha_x (nm/V)"=w4805:dbl, "T1 kappa_x (pN/nm)"=w4804:dbl)
        n3777 = Divide(x=w4811, y=w4813) -> (x/y=w4814:dbl)
        n3778 = To Long Integer(number=w4814) -> (32bit integer=w4812:i32)
        n3779 = Index Array(array=w4810, index=w4812) -> (element=w4797:dbl)
        n3780 = Multiply(x=w4805, y=w4804) -> (x*y=w4803:dbl)
        n3781 = Select(t=1, s=w4795, f=-1) -> (s? t:f=w4798:i32)
        n3782 = Divide(x=w4807, y=w4803) -> (x/y=w4802:dbl)
        n3783 = Multiply(x=w4798, y=w4797) -> (x*y=w4796:dbl)
        n3784 = Add(x=w4802, y=w4796) -> (x+y=w4801:dbl)
        n3785 = To Fixed-Point(number=w4801) -> (fixed-point=w4793:fxp<+/-,16,1>)  [unwired: 1 in]
        "Actual Setpoint" <- w4793
        n3786 = xnode "Read/Write Control"("FPGA VI Reference In"=w4794, "Trap Pos. FB SP"=w4793) -> ()  [unwired: 1 in, 2 out]
      }
    }
    n3787 = local read "All FB On/Off"() -> (w4419:bool)
    n3788 = case shown="True" w4419 {
      tunnel: w4420 -> [_ w4817]
      frame False {
      }
      frame True {
        n3789 = Divide(x=w4817, y=3276.7) -> (x/y=w4815:cluster{"Set 1":dbl, "Set 2":dbl})
        n3790 = Unbundle By Name(w4815) -> ("Set 1"=w4822:dbl, "Set 2"=w4821:dbl)
        n3791 = Greater?(x=w4822, y="Feedback Auto-Off threshold") -> (0:w4820:bool)
        n3792 = Greater?(x=w4821, y="Feedback Auto-Off threshold") -> (0:w4819:bool)
        n3793 = Or(x=w4820, y=w4819) -> (x .or. y?=w4818:bool)
        n3794 = case shown="True" w4818 {
          frame False {
          }
          frame True {
            n3795 = property on="All FB On/Off" class="Bool (strict)"("Val(Sgnl)"=FALSE) -> ()  [unwired: 2 in, 2 out]
          }
        }
      }
    }
    n3796 = flat-sequence "To save data" {
      tunnel: [w5923] -> w4777
      tunnel: [w5924] -> w4776
      tunnel: w4731 -> [w5917]
      tunnel: w4537 -> [w5921]
      tunnel: ["Save Calibration"] -> w4751
      tunnel: w4748 -> [w5920]
      tunnel: [w5913] -> w4747
      tunnel: [w5910] -> w4746
      tunnel: [w5907] -> w4745
      tunnel: w4730 -> [w5909]
      tunnel: w4672 -> [w5903]
      tunnel: [w5903] -> w4671
      tunnel: [w5895] -> w4646
      tunnel: [w5898] -> w4577
      tunnel: [w5897] -> w4576
      tunnel: [w5891] -> w4428
      tunnel: [w5887] -> w4412
      tunnel: w4777 -> [w6237]
      tunnel: w4776 -> [w6236]
      tunnel: w4578 -> [w6235]
      tunnel: w4751 -> [w6234]
      tunnel: w4747 -> [w6232]
      tunnel: w4746 -> [w6231]
      tunnel: w4745 -> [w6230]
      tunnel: w4654 -> [w6229]
      tunnel: w4680 -> [w6228]
      tunnel: w4671 -> [w6227]
      tunnel: w4646 -> [w6226]
      tunnel: w4435 -> [w6225]
      tunnel: w4481 -> [w6224]
      tunnel: w4577 -> [w6223]
      tunnel: w4576 -> [w6222]
      tunnel: w4575 -> [w6221]
      tunnel: w4503 -> [w6220]
      tunnel: w4426 -> [w6219]
      tunnel: w4428 -> [w6218]
      tunnel: w4412 -> [w6217]
      frame #0 {
        # "Changed by Ronen - we don't have a database so we disabled this"
        n3797 = Or(x="Start Saving", y="Start saving data + video") -> (x .or. y?=w5895:bool)
        n3798 = case shown="True" "Start saving data + video" {
          frame False {
          }
          frame True {
            n3799 = stacked-sequence {
              frame #0 {
                n3800 = local write "New Video File"(TRUE ("New Video File")) -> ()
              }
              frame #1 {
                n3801 = local write "Save Video"(TRUE ("Save Video")) -> ()
              }
            }
          }
        }
        n3802 = Or(x="Save N Sets", y=w5895) -> (x .or. y?=w5904:bool)
        n3803 = To Double Precision Float(number=w5920) -> (double precision float=w5914:dbl)
        n3804 = Build Array(w5904, "Save Calibration", w5917, w5909, "Flow Cal") -> (w5919:bool[])
        n3805 = Compound Arithmetic op=OR("Save Calibration", w5917, w5904, w5909, "Flow Cal") -> (w5922:bool)
        n3806 = Boolean Array To Number(Boolean array=w5919) -> (number=w5916:u32)
        n3807 = feedback #29(FALSE ("Save APD Data\nwith Trap Data")) -> (w5899:bool)
        n3808 = feedback #30(refnum<k0> refnum) -> (w5925:refnum<file>)
        n3809 = feedback #31(FALSE ("Save APD Data\nwith Trap Data")) -> (w5908:bool)
        n3810 = feedback #32(0) -> (w5927:i32)
        n3811 = feedback #33() -> (w5915:u32)  [unwired: 1 out]
        n3812 = feedback #34(refnum<k0> refnum) -> (w5892:refnum<file>)
        n3813 = feedback #35(refnum<k0> refnum) -> (w5901:refnum<file>)
        n3814 = feedback #36(refnum<k0> refnum) -> (w5888:refnum<file>)
        n3815 = feedback #37(refnum<k0> refnum) -> (w5911:refnum<file>)
        n3816 = case shown="True" w5922 {
          tunnel: [w5938 1] -> w5923
          tunnel: w5927 -> [w5940 _]
          tunnel: [w5939 w5972] -> w5924
          tunnel: w5925 -> [w5939 _]
          tunnel: w5921 -> [_ w5990]
          tunnel: w5914 -> [_ w5988]
          tunnel: w5916 -> [_ w5991]
          tunnel: [w5937 w5971] -> w5913
          tunnel: w5915 -> [w5937 _]
          tunnel: [w5936 w5969] -> w5910
          tunnel: w5911 -> [w5936 _]
          tunnel: [w5935 w5968] -> w5907
          tunnel: w5908 -> [w5935 _]
          tunnel: w5895 -> [_ w5966]
          tunnel: w5903 -> [_ w5965]
          tunnel: [w5934 w5958] -> w5897
          tunnel: w5901 -> [w5934 _]
          tunnel: [w5933 w5957] -> w5898
          tunnel: w5899 -> [w5933 _]
          tunnel: [w5932 w5943] -> w5891
          tunnel: w5892 -> [w5932 _]
          tunnel: [w5931 w5941] -> w5887
          tunnel: w5888 -> [w5931 _]
          frame False {
            n3817 = Increment(x=w5940) -> (x+1=w5938:i32)
          }
          frame True {
            w5942 = FALSE ("Start Saving")
            w5967 = 10.0  # File Version
            w5974 = FALSE ("prepend array or string size? (T)")
            w5973 = T41."big-endian, network order" ("byte order (0:big-endian, network order)")
            # "Ronen Changed the create file - changed data folder to c:\\Data"
            # "Save trap position\ndata"
            n3818 = local read "BD 1 Frequency 1 (MHz)"() -> (w5987:dbl)
            n3819 = local read "BD 2 Frequency 1 (MHz)"() -> (w5986:dbl)
            n3820 = local read "BD 1 Frequency 2 (MHz)"() -> (w5985:dbl)
            n3821 = local read "BD 2 Frequency 2 (MHz)"() -> (w5984:dbl)
            n3822 = local read "BD 1 Frequency 3 (MHz)"() -> (w5983:dbl)
            n3823 = local read "BD 2 Frequency 3 (MHz)"() -> (w5982:dbl)
            n3824 = Array Size(array=w5965) -> (size(s)=w5964:i32)
            n3825 = To Double Precision Float(number=w5964) -> (double precision float=w5963:dbl)
            n3826 = local write "Flow Cal"(w5942) -> ()
            n3827 = local write "Save Calibration"(w5942) -> ()
            n3828 = local write "Start Saving"(w5942) -> ()
            n3829 = Build Array("Save APD Data\nwith Trap Data", "Save Trap Pos. Data") -> (w5960:bool[])
            n3830 = Boolean Array To Number(Boolean array=w5960) -> (number=w5959:u32)
            n3831 = Build Array(w5987, w5986, w5985, w5984, w5983, w5982) -> (w5981:dbl[])
            n3832 = case shown="16" w5991 {
              tunnel: w5990 -> [w6091 w6118 w6134 w6172 w6209]
              tunnel: w5963 -> [w6096 w6125 w6154 w6191 w6214]
              tunnel: w5988 -> [w6095 w6124 w6153 w6190 w6213]
              tunnel: [w6092 w6120 w6145 w6182 w6210] -> w5979
              tunnel: [w6083 "Cal sets to save" w6135 w6173 w6196] -> w5971
              tunnel: w5981 -> [w6093 w6121 w6147 w6184 w6211]
              tunnel: "Save APD Data\nwith Trap Data" -> [w6090 w6107 w6131 w6170 w6208]
              tunnel: [w6090 w6105 w6131 w6170 w6208] -> w5968
              tunnel: w5967 -> [w6086 w6114 w6129 w6168 w6204]
              tunnel: w5966 -> [w6085 _ _ _ _]
              tunnel: [w6076 w6113 w6128 w6158 w6203] -> w5957
              tunnel: "Save Trap Pos. Data" -> [w6076 w6112 w6128 w6158 w6203]
              tunnel: w5959 -> [w6075 w6111 w6127 w6157 w6202]
              frame 1, Default {
                # "timeseries"
                n3833 = case shown="True" "Profile" {
                  tunnel: [w6099 w6103] -> w6080
                  tunnel: [w6099 w6102] -> w6079
                  tunnel: [w6099 w6101] -> w6078
                  tunnel: [w6099 w6100] -> w6077
                  frame False {
                    w6099 = 0.0 ("f")
                  }
                  frame True {
                    n3834 = local read "Current Position"() -> (w6104:cluster{dbl, dbl, dbl})
                    n3835 = local read "Y change (mm)"() -> (w6100:dbl)
                    n3836 = Unbundle(w6104) -> (w6103:dbl, w6102:dbl, w6101:dbl)
                  }
                }
                n3837 = local read "Save ave N"() -> (w6098:dbl)
                n3838 = Multiply(x=w6098, y=w6091) -> (x*y=w6097:dbl)
                n3839 = To Double Precision Float(number=w6075) -> (double precision float=w6089:dbl)
                n3840 = Build Array(w6086, w6091, w6097, w6096, w6095, 0.0 ("f")) -> (w6094:dbl[])
                n3841 = Build Array(w6089, w6080, w6079, w6078, w6077) -> (w6087:dbl[])
                n3842 = Select(t=u32 4000000000, s=w6085, f="N sets to save") -> (s? t:f=w6083:u32)
                n3843 = Build Array (concatenate)(w6094, w6093, w6087) -> (w6092:dbl[])
              }
              frame 2 {
                w6116 = 0.0 ("f")
                w6106 = FALSE ("Save APD Data\nwith Trap Data")
                # "For diagnostics save trap position\ndata during cal"
                # "calibration"
                n3844 = Boolean To (0,1)(Boolean=w6106) -> (0, 1=w6110:i16)
                n3845 = Select(t=w6107, s="Save trap pos with cal", f=w6106) -> (s? t:f=w6105:bool)
                n3846 = Select(t=w6112, s="Save trap pos with cal", f=w6106) -> (s? t:f=w6113:bool)
                n3847 = Select(t=w6111, s="Save trap pos with cal", f=w6110) -> (s? t:f=w6109:u32)
                n3848 = To Double Precision Float(number=w6109) -> (double precision float=w6117:dbl)
                n3849 = Build Array(w6114, w6118, w6118, w6125, w6124, 1.0 ("t")) -> (w6122:dbl[])
                n3850 = Build Array(w6117, w6116, w6116, w6116, w6116) -> (w6115:dbl[])
                n3851 = Build Array (concatenate)(w6122, w6121, w6115) -> (w6120:dbl[])
                "Calibrating Trap..." <- TRUE ("Calibrating...")
              }
              frame 4 {
                w6132 = 0.0 ("f")
                # "scan dir (x/y = 0/1)"
                # "cycles/step"
                # "n scans (f/b)"
                # "steps"
                # "freq. range"
                # "AOD raster scan"
                n3852 = local read "Number of F/B Scans (AOD)"() -> (w6139:u16)
                n3853 = local read "Cycles/step (AOD)"() -> (w6141:u64)
                n3854 = local read "Scan Range (MHz)"() -> (w6144:dbl)
                n3855 = local read "Scan steps (AOD)"() -> (w6143:u64)
                n3856 = local read "Scan BD"() -> (w6151:bool)
                n3857 = local read "Save ave N"() -> (w6156:dbl)
                n3858 = Boolean To (0,1)(Boolean=w6151) -> (0, 1=w6150:i16)
                n3859 = To Double Precision Float(number=w6139) -> (double precision float=w6138:dbl)
                n3860 = To Double Precision Float(number=w6143) -> (double precision float=w6142:dbl)
                n3861 = To Double Precision Float(number=w6141) -> (double precision float=w6140:dbl)
                n3862 = To Double Precision Float(number=w6150) -> (double precision float=w6149:dbl)
                n3863 = Multiply(x=w6156, y=w6134) -> (x*y=w6155:dbl)
                n3864 = To Double Precision Float(number=w6127) -> (double precision float=w6133:dbl)
                n3865 = Build Array(w6133, w6132, w6132, w6132, w6132) -> (w6130:dbl[])
                n3866 = local read "N sets should be saved"() -> (w6136:dbl)
                n3867 = Build Array(w6149, w6144, w6142, w6140, w6138) -> (w6146:dbl[])
                n3868 = Build Array(w6129, w6134, w6155, w6154, w6153, 2.0 ("t")) -> (w6148:dbl[])
                n3869 = Round Toward +Infinity(x=w6136) -> (ceil(x): smallest int >= x=w6137:dbl)
                n3870 = Build Array (concatenate)(w6148, w6147, w6130, w6146) -> (w6145:dbl[])
                n3871 = To Unsigned Long Integer(number=w6137) -> (unsigned 32bit integer=w6135:u32)
              }
              frame 8 {
                w6165 = 0.0 ("f")
                # "MCL raster scan"
                n3872 = local read "Number of scans (MCL)"() -> (w6160:u64)
                n3873 = local read "2D or 1D Scan"() -> (w6162:bool)
                n3874 = local read "Scan lines (y)"() -> (w6159:u64)
                n3875 = local read "Scan Range (V)\n(of steps)"() -> (w6181:dbl)
                n3876 = local read "Fast Scan Dir"() -> (w6188:bool)
                n3877 = local read "Cycles/step (MCL)"() -> (w6178:u64)
                n3878 = local read "Scan steps (MCL)"() -> (w6180:u64)
                n3879 = Select(t=w6159, s=w6162, f=w6160) -> (s? t:f=w6161:u64)
                n3880 = Boolean To (0,1)(Boolean=w6162) -> (0, 1=w6164:i16)
                n3881 = local read "Save ave N"() -> (w6193:dbl)
                n3882 = local read "Initial X"() -> (w6167:dbl)
                n3883 = local read "Initial Y"() -> (w6166:dbl)
                n3884 = To Double Precision Float(number=w6164) -> (double precision float=w6163:dbl)
                n3885 = Boolean To (0,1)(Boolean=w6188) -> (0, 1=w6187:i16)
                n3886 = To Double Precision Float(number=w6161) -> (double precision float=w6176:dbl)
                n3887 = To Double Precision Float(number=w6180) -> (double precision float=w6179:dbl)
                n3888 = To Double Precision Float(number=w6178) -> (double precision float=w6177:dbl)
                n3889 = To Double Precision Float(number=w6187) -> (double precision float=w6186:dbl)
                n3890 = Multiply(x=w6193, y=w6172) -> (x*y=w6192:dbl)
                n3891 = To Double Precision Float(number=w6157) -> (double precision float=w6171:dbl)
                n3892 = local read "N sets should be saved (MCL)"() -> (w6174:dbl)
                n3893 = Build Array(w6171, w6163, w6165, w6165, w6165) -> (w6169:dbl[])
                n3894 = Build Array(w6186, w6181, w6179, w6177, w6176, w6167, w6166) -> (w6183:dbl[])
                n3895 = Build Array(w6168, w6172, w6192, w6191, w6190, 3.0 ("t")) -> (w6185:dbl[])
                n3896 = Round Toward +Infinity(x=w6174) -> (ceil(x): smallest int >= x=w6175:dbl)
                n3897 = Build Array (concatenate)(w6185, w6184, w6169, w6183) -> (w6182:dbl[])
                n3898 = To Unsigned Long Integer(number=w6175) -> (unsigned 32bit integer=w6173:u32)
              }
              frame 16 {
                w6195 = 0.0
                # "Flow calibration - added by Ronen: Number\nof saved sets is distance (1 mm) divided by \nspeed +1.5 spare second divided by the time of\nset measurement, 0.2 sec for 2 set interlace"
                # "timeseries"
                n3899 = local read "Save ave N"() -> (w6216:dbl)
                n3900 = Reciprocal(x=0.0) -> (1/x=w6201:dbl)
                n3901 = Add(x=w6201, y=1.5) -> (x+y=w6199:dbl)
                n3902 = Multiply(x=w6216, y=w6209) -> (x*y=w6215:dbl)
                n3903 = Divide(x=w6199, y=0.2) -> (x/y=w6197:dbl)
                n3904 = To Double Precision Float(number=w6202) -> (double precision float=w6207:dbl)
                n3905 = To Unsigned Long Integer(number=w6197) -> (unsigned 32bit integer=w6196:u32)
                n3906 = Build Array(w6204, w6209, w6215, w6214, w6213, 4.0 ("f")) -> (w6212:dbl[])
                n3907 = Build Array(w6207, w6195, w6195, w6195, w6195) -> (w6205:dbl[])
                n3908 = Build Array (concatenate)(w6212, w6211, w6205) -> (w6210:dbl[])
              }
            }
            n3909 = local read "Index"() -> (w5996:dbl)
            n3910 = call "Create new save file.vi"("Insert"="", "Ext"=".dat", "Index In"=w5996) -> ("Path Out"=w5945:path, "Index Out"=w5970:dbl)
            n3911 = local write "Save file name"(w5945) -> ()
            n3912 = local write "Index"(w5970) -> ()
            n3913 = local write "Save index"(w5970) -> ()
            n3914 = case shown="True" "Save Event Log?" {
              tunnel: w5945 -> [_ w6010]
              tunnel: [refnum<k0> refnum w6009] -> w5943
              frame False {
              }
              frame True {
                (unwired) FALSE ("prepend array or string size? (T)")
                n3915 = Path To String(path=w6010) -> (string=w6021:string)
                n3916 = String Length(string=w6021) -> (length=w6020:i32)
                n3917 = Subtract(x=w6020, y=4) -> (x-y=w6018:i32)
